vi "sub_SDR_siso_RemovePilots.vi"(8 "Symbols per pilot":i32, 9 "Payload Symbols":i32, 10 "Array in":cdb[](array[numeric])) -> (1 "Pilots SNR":dbl, 2 "Array Out":cdb[](array[numeric]))   [LabVIEW 2012]
uses:
  <vilib>/Analysis/NI_AALBase.lvlib
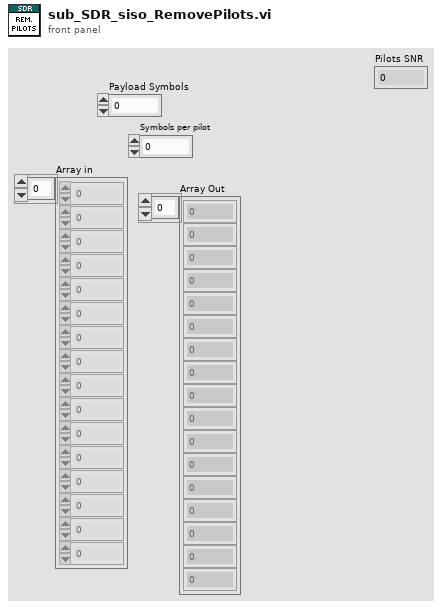
[diagram p1: front panel]
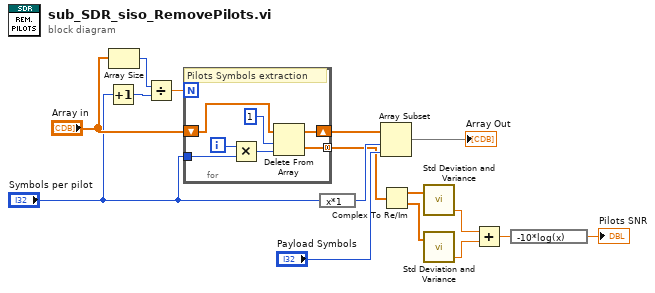
[diagram p0: block diagram]
diagram:
  n1 = Increment(x="Symbols per pilot") -> (x+1=w9:i32)
  n2 = Array Size(array="Array in") -> (size(s)=w12:i32)
  n3 = Divide(x=w12, y=w9) -> (x/y=w13:dbl)
  n4 = for {
    N: w13 -> [_]
    shift-right: [w22] -> w11
    shift-left: "Array in" -> [w23]
    tunnel: "Symbols per pilot" -> [w18]
    tunnel: [w17] -> w1 mode=concatenating
    i -> [w20]
    # "Pilots Symbols extraction"
    n5 = Multiply(x=w20, y=w18) -> (x*y=w19:i32)
    n6 = Delete From Array(array=w23, length=1, index=w19) -> (deleted portion=w17:cdb[], array with subset deleted=w22:cdb[])
  }
  n7 = expression code="x*1"("Symbols per pilot") -> (w16:i32)
  n8 = Array Subset "Array Subset"(array=w11, index=w16, length="Payload Symbols") -> (→"Array Out":cdb[])
  n9 = Complex To Re/Im(x + iy=w1) -> (x=w7:dbl[], y=w6:dbl[])
  n10 = call <vilib>:"Std Deviation and Variance.vi"("X"=w7) -> ("variance"=w5:dbl)  [unwired: 1 in, 2 out]
  n11 = call <vilib>:"Std Deviation and Variance.vi"("X"=w6) -> ("variance"=w4:dbl)  [unwired: 1 in, 2 out]
  n12 = Add(x=w5, y=w4) -> (x+y=w2:dbl)
  n13 = expression code="-10*log(x)"(w2) -> (→"Pilots SNR":dbl)
